vi "Open All Gyros.vi"   [LabVIEW 2016, in "Apple Pi Gyro Library.lvlib"]
uses:
  Apple Pi Gyro Library.lvlib
  <vilib>/Rock Robotics/SystemInterfaces/spilib/spi_bus.ctl
  <vilib>/Rock Robotics/SystemInterfaces/AI/FPGA_AIGyroChannel.ctl
  NavX/NI WPI/WPI_SerialPort_USB.ctl
  <vilib>/Rock Robotics/WPI/Gyro/WPI_GyroAnalogOpen.vi
  NavX/navX Library v2/IO/Open/Z900_navX_Open_Serial.vi
  ADI MXP IMU/ADI MXP IMU/FRC_ADIS16448_IMU.lvlib
  SimpleGyro ADXRS453/SimpleGyro.lvlib
  NavX/navX Library v2/navX Library v2.lvlib
  NavX/NI WPI/NI WPI Serial USB.lvlib
panel:
  # "Throw me into Begin.vi\n\nCheck where everything\n is plugged in\n\ndefault set up allows everything\n to run at the saame time"
  # "All done :D"
types:
  T1 = typedef "NI WPI Serial USB.lvlib/WPI_SerialPort_USB.ctl" = enum16{"Onboard RS-232", "MXP TTL", "USB"}
  T2 = typedef "FPGA_AIGyroChannel.ctl" = enum8{"AI 0", "AI 1", "Invalid"}
  T3 = typedef "spi_bus.ctl" = enum16{"SPI On-Board, CS0", "SPI On-Board, CS1", "SPI On-Board, CS2", "SPI On-Board, CS3", "SPI MXP", "Invalid"}
  T4 = typedef "Apple Pi Gyro Library.lvlib/SimpleGyro.lvlib/WPI_SimpleGyroDevRef.ctl" = cluster{"DevStatus":errorcluster, "Handle":i32, "SPI Bus":T3, "Device Found":bool, "Sample Rate":dbl}
  T5 = typedef "WPI_GyroDevRef.ctl" = cluster{"DevStatus":errorcluster, "Analog Channel":T6, "Offset":dbl, "Gain (VoltsPerDegree/Second)":dbl, "Gyro Type":enum16{"Analog", "XRS450"}, "Handle":i32, "SPI Bus":T3, "Device Found":bool, "Sample Rate":dbl, "Calibrate On Open":bool}
  T6 = typedef "FPGA_AIChannel.ctl" = enum8{"AI 0", "AI 1", "AI 2", "AI 3", "AI MXP 0", "AI MXP 1", "AI MXP 2", "AI MXP 3", "Invalid"}
  T7 = typedef "Apple Pi Gyro Library.lvlib/navX Library v2.lvlib/Z900_navX_DeviceTypeDef.ctl" = cluster{"Interface":cluster{"Protocol":T8, "Update Rate (4Hz-100Hz)":u8, "navX Open TypeDef":variant}, "Notify Packet":refnum<notifier>, "Loop VI Refnum":refnum<vi>, "Ready to Close Occurrence Refnum":refnum<k4>}
  T8 = typedef "Apple Pi Gyro Library.lvlib/navX Library v2.lvlib/Z900_navX_ProtocolTypeDef.ctl" = enum16{"SERIAL", "I2C", "SPI"}
  T9 = typedef "Apple Pi Gyro Library.lvlib/FRC_ADIS16448_IMU.lvlib/WPI_IMU_ADIS16448_InterruptDevRef.ctl" = cluster{"ADI IMU DevRef":T10, "InterruptRef":T11}
  T10 = typedef "Apple Pi Gyro Library.lvlib/FRC_ADIS16448_IMU.lvlib/WPI_IMU_ADIS16448_IMUDevRef.ctl" = cluster{"DevStatus":errorcluster, "Handle":i32, "SPI Bus":T3, "Device Found":bool, "Device Ready":bool, "Yaw Axis":enum16{"X", "Y", "Z"}, "AHRS Algorithm":enum16{"Complementary", "Madgwick"}, "Serial":u16, "Lot ID 2":u16, "Lot ID 1":u16, "Product ID":u16}
  T11 = typedef "WPI_InterruptRef.ctl" = cluster{"DevStatus":errorcluster, "InterruptIndex":T12}
  T12 = typedef "FPGA_InterruptIndex.ctl" = enum8{"0", "1", "2", "3", "4", "5", "6", "7", "Invalid"}
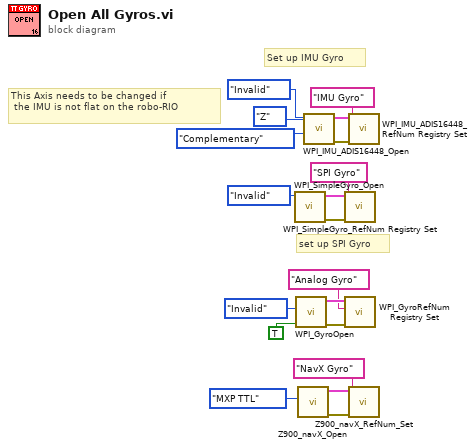
[diagram p0: block diagram]
diagram:
  # "set up SPI Gyro"
  # "This Axis needs to be changed if\n the IMU is not flat on the robo-RIO"
  # "Set up IMU Gyro"
  n1 = call "WPI_SimpleGyro_Open.vi"("SPI Chip Select"=spi_bus."Invalid") -> ("error out"=w14:errorcluster, "SimpleGyroDevRef"=w13:T4)  [unwired: 9 in]
  n2 = call-poly <vilib>:"WPI_GyroOpen.vi"("Calibrate On Open"=TRUE, "Analog Channel"=FPGA_AIGyroChannel."Invalid") -> ("error out"=w9:errorcluster, "GyroDevRef"=w8:T5)  [unwired: 7 in, 1 out]
  n3 = call-poly "Z900_navX_Open.vi"("Serial Port"=WPI_SerialPort_USB."MXP TTL") -> ("error out"=w3:errorcluster, "navX Device"=w2:T7)  [unwired: 9 in]
  n4 = call "WPI_IMU_ADIS16448_Open.vi"("AHRS Algorithm"=enum16{"Complementary", "Madgwick"}."Complementary", "Yaw Axis"=enum16{"X", "Y", "Z"}."Z", "SPI Chip Select"=spi_bus."Invalid") -> ("error out"=w19:errorcluster, "ADI IMU Interrupt DevRef"=w18:T9)  [unwired: 7 in]
  n5 = call "WPI_SimpleGyro_RefNum Registry Set.vi"("error in (no error)"=w14, "refnum name"="SPI Gyro", "SimpleGyroDevRef"=w13) -> ()  [unwired: 7 in, 2 out]
  n6 = call <vilib>:"WPI_GyroRefNum Registry Set.vi"("error in (no error)"=w9, "refnum name"="Analog Gyro", "GyroDevRef"=w8) -> ()  [unwired: 7 in, 2 out]
  n7 = call "WPI_IMU_ADIS16448_RefNum Registry Set.vi"("error in (no error)"=w19, "refnum name"="IMU Gyro", "ADI IMU Interrupt DevRef"=w18) -> ()  [unwired: 7 in, 2 out]
  n8 = call "Z900_navX_RefNum_Set.vi"("error in (no error)"=w3, "refnum name"="NavX Gyro", "navX Device"=w2) -> ()  [unwired: 7 in, 2 out]
